vi "PathPlanner_Waypoint_Equals.vi"(9 "Other Waypoint":T1={"prevControl"={"X"=0.0, "Y"=1.0}, "anchor"={"X"=0.0, "Y"=0.0}, "nextControl"={"X"=0.0, "Y"=0.0}, "PrevExists"=FALSE, "NextExists"=FALSE} {"nextControl"."Y" format="%14.3f"; "nextControl"."X" format="%14.3f"; "anchor"."Y" format="%14.3f"; "anchor"."X" format="%14.3f"; "prevControl"."Y" format="%14.3f"; "prevControl"."X" format="%14.3f"}, 11 "PathPlannerWaypoint":T1={"prevControl"={"X"=0.0, "Y"=1.0}, "anchor"={"X"=0.0, "Y"=0.0}, "nextControl"={"X"=0.0, "Y"=0.0}, "PrevExists"=FALSE, "NextExists"=FALSE} {"nextControl"."Y" format="%14.3f"; "nextControl"."X" format="%14.3f"; "anchor"."Y" format="%14.3f"; "anchor"."X" format="%14.3f"; "prevControl"."Y" format="%14.3f"; "prevControl"."X" format="%14.3f"}) -> (3 "Equal":bool)   [LabVIEW 2019, in "PathPlanner24.lvlib"]
doc: "Determine if two rotation targets are equal\n\nInputs: \n - RotationTarget - cluster - defined rotation target data structure\n - OtherRotationTarget - cluster - defined rotation target data structure\n\nOutputs:\n - Equal - boolean - TRUE if both rotation targets are the same"
uses:
  <vilib>/Rock Robotics/WPI/ThirdParty/JAS_Junk/TrajLib/Util_CalcDist.vi
  PathPlanner24.lvlib
  <vilib>/Rock Robotics/WPI/ThirdParty/JAS_Junk/TrajLib/Trajectory_Library.lvlib
  <vilib>/Rock Robotics/WPI/ThirdParty/JAS_Junk/TrajLib/TypeDef/TRANSLATION2D.ctl
  TypeDef/PathPlannerWaypoint.ctl
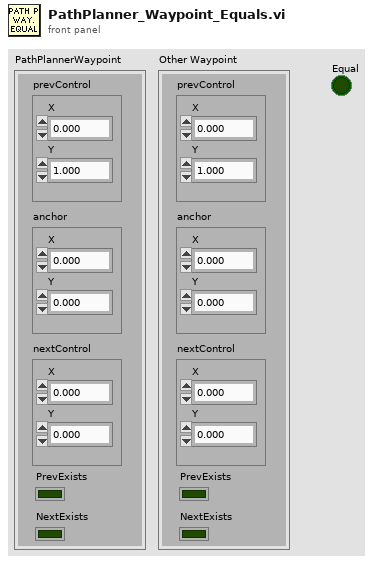
[diagram p1: front panel]
types:
  T1 = typedef "PathPlanner24.lvlib/PathPlannerWaypoint.ctl" = cluster{"prevControl":T2, "anchor":T2, "nextControl":T2, "PrevExists":bool, "NextExists":bool}
  T2 = typedef "Trajectory_Library.lvlib/TRANSLATION2D.ctl" = cluster{"X":dbl, "Y":dbl}
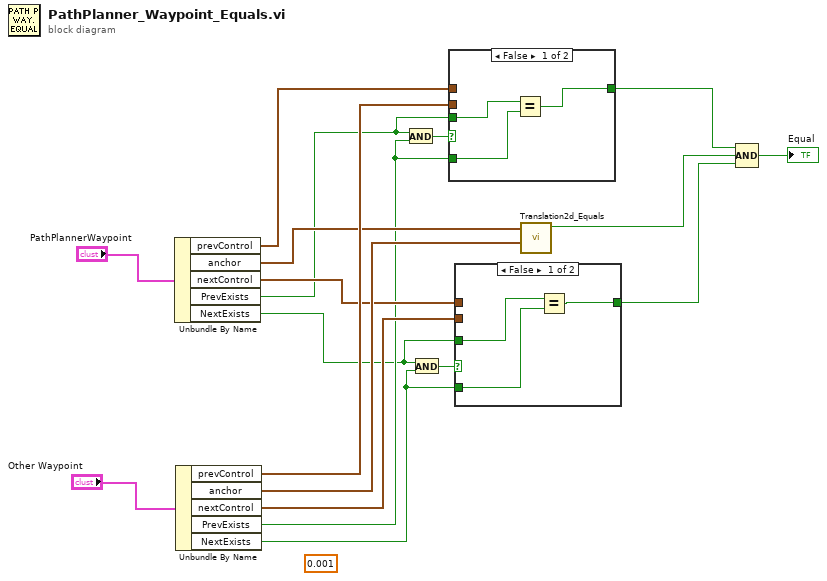
[diagram p0: block diagram]
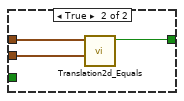
[diagram p2: hidden frame]
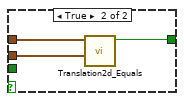
[diagram p3: hidden frame]
diagram:
  (unwired) 0.001 ("y")
  n1 = Unbundle By Name("PathPlannerWaypoint") -> ("prevControl"=w15:T2, "anchor"=w12:T2, "nextControl"=w8:T2, "PrevExists"=w5:bool, "NextExists"=w3:bool)
  n2 = Unbundle By Name("Other Waypoint") -> ("prevControl"=w14:T2, "anchor"=w11:T2, "nextControl"=w7:T2, "PrevExists"=w4:bool, "NextExists"=w2:bool)
  n3 = And(x=w5, y=w4) -> (x .and. y?=w16:bool)
  n4 = And(x=w3, y=w2) -> (x .and. y?=w13:bool)
  n5 = case shown="False" w16 {
    tunnel: w15 -> [_ w24]
    tunnel: w14 -> [_ w23]
    tunnel: [w19 w22] -> w10
    tunnel: w5 -> [w21 _]
    tunnel: w4 -> [w20 _]
    frame False {
      n6 = Equal?(x=w21, y=w20) -> (x = y?=w19:bool)
    }
    frame True {
      n7 = call <vilib>:"Translation2d_Equals.vi"("other Translation"=w23, "In Translation"=w24) -> ("Equals"=w22:bool)  [unwired: 9 in]
    }
  }
  n8 = case shown="False" w13 {
    tunnel: w8 -> [_ w30]
    tunnel: w7 -> [_ w29]
    tunnel: [w25 w28] -> w6
    tunnel: w3 -> [w27 _]
    tunnel: w2 -> [w26 _]
    frame False {
      n9 = Equal?(x=w27, y=w26) -> (x = y?=w25:bool)
    }
    frame True {
      n10 = call <vilib>:"Translation2d_Equals.vi"("other Translation"=w29, "In Translation"=w30) -> ("Equals"=w28:bool)  [unwired: 9 in]
    }
  }
  n11 = call <vilib>:"Translation2d_Equals.vi"("other Translation"=w11, "In Translation"=w12) -> ("Equals"=w9:bool)  [unwired: 9 in]
  n12 = Compound Arithmetic op=AND(w10, w9, w6) -> (→"Equal":bool)
